vi "자동차세차기.vi"() -> ()   [LabVIEW 2018]
uses:
  Control/Wash Options.ctl
  Control/Car Position Control.ctl
  Control/Car Wash Indicators.ctl
  Control/WashState.ctl
panel:
  in  "Stop":bool
  out "경과 시간":dbl format="%#.2g"
  out "세차 인디케이터":T1
  in  "자동차 위치 슬라이더":T2 scale=0.0..4.0
  out "세차기 입구":bool
  in  "시작":bool
  in  "세차 옵션":T3
  # "입구 콘솔"
  # "세차 디스플레이"
  # "자동차 위치 시뮬레이션"
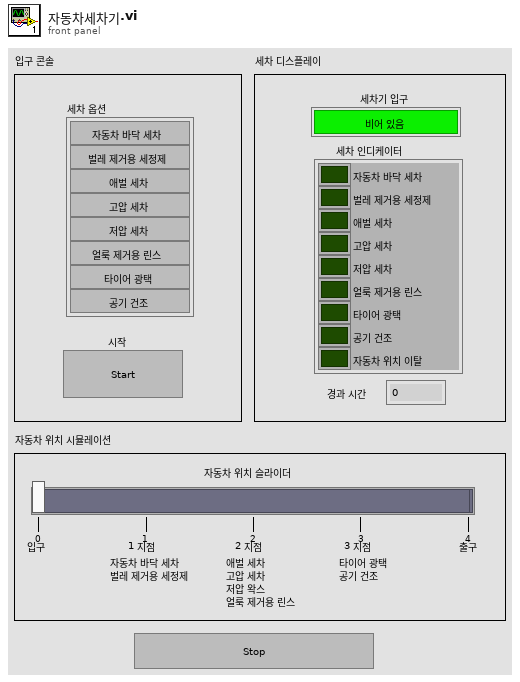
[diagram p1: front panel]
types:
  T1 = typedef "Car Wash Indicators.ctl" = cluster{"자동차 바닥 세차":bool, "벌레 제거용 세정제":bool, "애벌 세차":bool, "고압 세차":bool, "저압 세차":bool, "얼룩 제거용 린스":bool, "타이어 광택":bool, "공기 건조":bool, "자동차 위치 이탈":bool}
  T2 = typedef "Car Position Control.ctl" = i32
  T3 = typedef "Wash Options.ctl" = cluster{"Under Body Wash":bool, "Bug Remover":bool, "Pre-Soak":bool, "High Pressure Wash":bool, "Low Pressure Wax":bool, "Spot Free Rinse":bool, "Tire Shine Foam":bool, "Air Dry":bool}
  T4 = typedef "WashState.ctl" = enum16{"Initialize", "Ready", "Under Body Wash", "Bug Remover", "Pre-Soak", "High Pressure Wash", "Low Pressure Wax", "Spot Free Rinse", "Tire Shine Foam", "Air Dry", "Stop", "Exit"}
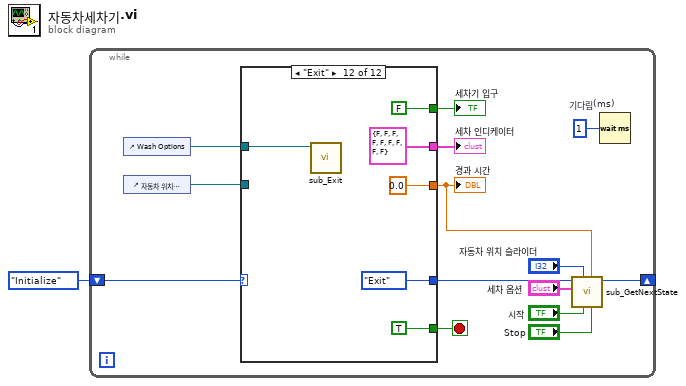
[diagram p0: block diagram]
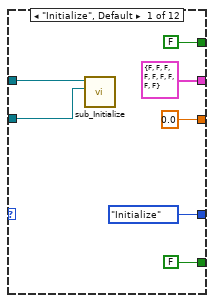
[diagram p2: hidden frame]
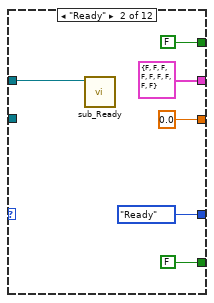
[diagram p3: hidden frame]
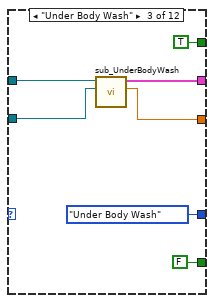
[diagram p4: hidden frame]
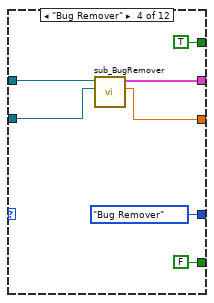
[diagram p5: hidden frame]
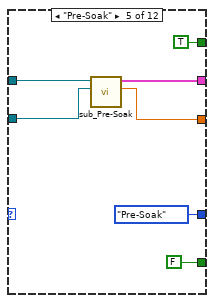
[diagram p6: hidden frame]
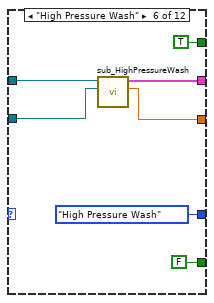
[diagram p7: hidden frame]
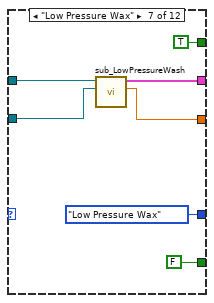
[diagram p8: hidden frame]
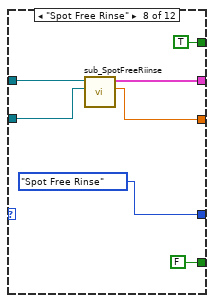
[diagram p9: hidden frame]
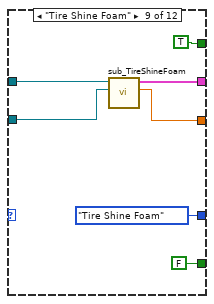
[diagram p10: hidden frame]
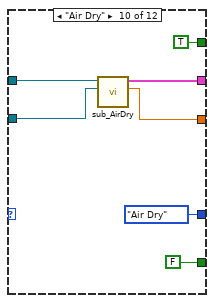
[diagram p11: hidden frame]
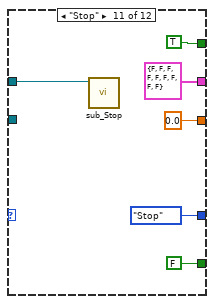
[diagram p12: hidden frame]
diagram:
  n1 = while {
    shift-right: [w13] -> _
    shift-left: WashState."Initialize" ("WashState") -> [w15]
    stop <- w11 stop-if-true
    n2 = control-ref of="Wash Options"() -> (w6:refnum<vi>)
    n3 = control-ref of="자동차 위치 슬라이더"() -> (w5:refnum<vi>)
    n4 = case shown="\"Exit\"" w15 {
      tunnel: [WashState."Initialize" ("CurrentState") WashState."Ready" ("CurrentState") WashState."Under Body Wash" ("CurrentState") WashState."Bug Remover" ("CurrentState") WashState."Pre-Soak" ("CurrentState") WashState."High Pressure Wash" ("CurrentState") WashState."Low Pressure Wax" ("CurrentState") WashState."Spot Free Rinse" ("WashState") WashState."Tire Shine Foam" ("CurrentState") WashState."Air Dry" ("CurrentState") WashState."Stop" ("CurrentState") WashState."Exit" ("CurrentState")] -> w14
      tunnel: [FALSE FALSE FALSE FALSE FALSE FALSE FALSE FALSE FALSE FALSE FALSE TRUE] -> w11
      tunnel: w6 -> [w17 w23 w30 w37 w44 w51 w58 w66 w72 w79 w85 w91]
      tunnel: w5 -> [w16 _ w29 w36 w43 w50 w57 w65 w71 w78 _ _]
      tunnel: [FALSE ("Wash Entry") FALSE ("Wash Entry") TRUE ("Wash Entry") TRUE ("Wash Entry") TRUE ("Wash Entry") TRUE ("Wash Entry") TRUE ("Wash Entry") TRUE ("Wash Entry") TRUE ("Wash Entry") TRUE ("Wash Entry") TRUE ("Wash Entry") FALSE ("Wash Entry")] -> w4
      tunnel: [T1 {"자동차 바닥 세차"=FALSE, "벌레 제거용 세정제"=FALSE, "애벌 세차"=FALSE, "고압 세차"=FALSE, "저압 세차"=FALSE, "얼룩 제거용 린스"=FALSE, "타이어 광택"=FALSE, "공기 건조"=FALSE, "자동차 위치 이탈"=FALSE} ("Wash Indicators") T1 {"자동차 바닥 세차"=FALSE, "벌레 제거용 세정제"=FALSE, "애벌 세차"=FALSE, "고압 세차"=FALSE, "저압 세차"=FALSE, "얼룩 제거용 린스"=FALSE, "타이어 광택"=FALSE, "공기 건조"=FALSE, "자동차 위치 이탈"=FALSE} ("Wash Indicators") w32 w39 w46 w53 w60 w68 w74 w81 T1 {"자동차 바닥 세차"=FALSE, "벌레 제거용 세정제"=FALSE, "애벌 세차"=FALSE, "고압 세차"=FALSE, "저압 세차"=FALSE, "얼룩 제거용 린스"=FALSE, "타이어 광택"=FALSE, "공기 건조"=FALSE, "자동차 위치 이탈"=FALSE} ("Wash Indicators") T1 {"자동차 바닥 세차"=FALSE, "벌레 제거용 세정제"=FALSE, "애벌 세차"=FALSE, "고압 세차"=FALSE, "저압 세차"=FALSE, "얼룩 제거용 린스"=FALSE, "타이어 광택"=FALSE, "공기 건조"=FALSE, "자동차 위치 이탈"=FALSE} ("Wash Indicators")] -> w3
      tunnel: [0.0 ("Elapsed Time (sec)") 0.0 ("Elapsed Time (sec)") w31 w38 w45 w52 w59 w67 w73 w80 0.0 ("Elapsed Time (sec)") 0.0 ("Elapsed Time (sec)")] -> w2
      frame "Initialize", Default {
        n5 = call "sub_Initialize.vi"("Car Position Slider"=w16, "Wash Options"=w17) -> ()  [unwired: 9 in, 1 out]
      }
      frame "Ready" {
        n6 = call "sub_Ready.vi"("Wash Options"=w23) -> ()  [unwired: 10 in, 1 out]
      }
      frame "Under Body Wash" {
        n7 = call "sub_UnderBodyWash.vi"("Car Position Slider"=w29, "Wash Options"=w30) -> ("Elapsed Time (sec)"=w31:dbl, "Wash Indicators"=w32:T1)  [unwired: 7 in, 1 out]
      }
      frame "Bug Remover" {
        n8 = call "sub_BugRemover.vi"("Car Position Slider"=w36, "Wash Options"=w37) -> ("Elapsed Time (sec)"=w38:dbl, "Wash Indicators"=w39:T1)  [unwired: 7 in, 1 out]
      }
      frame "Pre-Soak" {
        n9 = call "sub_Pre-Soak.vi"("Car Position Slider"=w43, "Wash Options"=w44) -> ("Elapsed Time (sec)"=w45:dbl, "Wash Indicators"=w46:T1)  [unwired: 7 in, 1 out]
      }
      frame "High Pressure Wash" {
        n10 = call "sub_HighPressureWash.vi"("Car Position Slider"=w50, "Wash Options"=w51) -> ("Elapsed Time (sec)"=w52:dbl, "Wash Indicators"=w53:T1)  [unwired: 7 in, 1 out]
      }
      frame "Low Pressure Wax" {
        n11 = call "sub_LowPressureWash.vi"("Car Position Slider"=w57, "Wash Options"=w58) -> ("Elapsed Time (sec)"=w59:dbl, "Wash Indicators"=w60:T1)  [unwired: 7 in, 1 out]
      }
      frame "Spot Free Rinse" {
        n12 = call "sub_SpotFreeRiinse.vi"("Car Position Slider"=w65, "Wash Options"=w66) -> ("Elapsed Time (sec)"=w67:dbl, "Wash Indicators"=w68:T1)  [unwired: 7 in, 1 out]
      }
      frame "Tire Shine Foam" {
        n13 = call "sub_TireShineFoam.vi"("Car Position Slider"=w71, "Wash Options"=w72) -> ("Elapsed Time (sec)"=w73:dbl, "Wash Indicators"=w74:T1)  [unwired: 7 in, 1 out]
      }
      frame "Air Dry" {
        n14 = call "sub_AirDry.vi"("Car Position Slider"=w78, "Wash Options"=w79) -> ("Elapsed Time (sec)"=w80:dbl, "Wash Indicators"=w81:T1)  [unwired: 7 in, 1 out]
      }
      frame "Stop" {
        n15 = call "sub_Stop.vi"("Wash Options"=w85) -> ()  [unwired: 10 in, 1 out]
      }
      frame "Exit" {
        n16 = call "sub_Exit.vi"("Wash Options"=w91) -> ()  [unwired: 10 in, 1 out]
      }
    }
    "세차 인디케이터" <- w3
    "경과 시간" <- w2
    "세차기 입구" <- w4
    n17 = call "sub_GetNextState.vi"("Stop"="Stop", "Elapsed Time (sec)"=w2, "Start"="시작", "Car Position Slider"="자동차 위치 슬라이더", "Wash Options"="세차 옵션", "CurrentState"=w14) -> ("NextState"=w13:T4)  [unwired: 4 in, 1 out]
    n18 = Wait (ms) "기다림(ms)"(milliseconds to wait=u32 1 ("대기 시간 (ms)")) -> ()  [unwired: 1 out]
  }
